vi "Read Save_.vi"(8 "error in (no error)":errorcluster, 11 "Save Data MSG in":refnum<class "Save Data MSG.lvclass">) -> (0 "error out":errorcluster, 2 "Save?":bool, 3 "Save Data MSG out":refnum<class "Save Data MSG.lvclass">)   [LabVIEW 2014, in "Controller.lvlib" / "Save Data MSG.lvclass"]
uses:
  Save Data MSG.lvclass
  Save Data MSG.lvclass/Save Data MSG.ctl
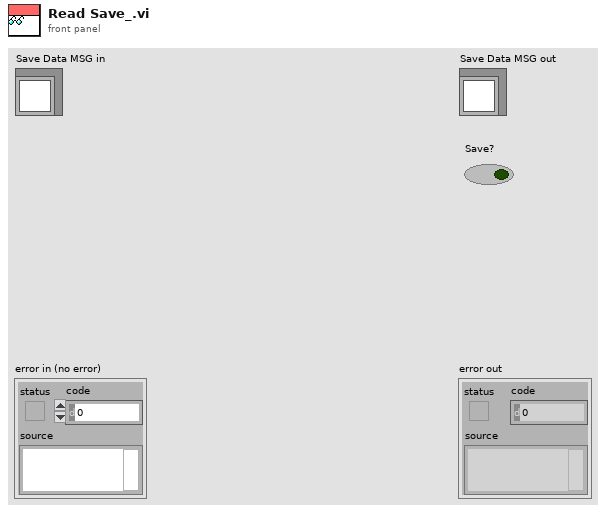
[diagram p1: front panel]
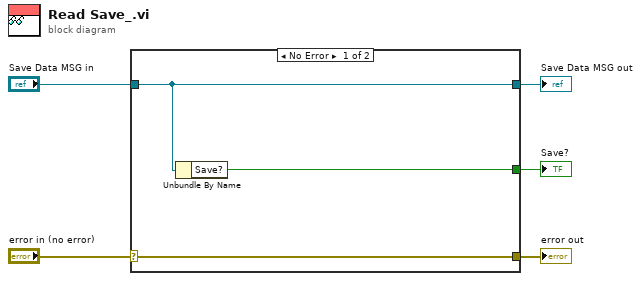
[diagram p0: block diagram]
diagram:
  n1 = case shown="No Error" "error in (no error)" {
    selector: "error in (no error)" -> [w8 w9]
    tunnel: [w8 w9] -> w4
    tunnel: [w7 w10] -> w2
    tunnel: "Save Data MSG in" -> [w7 w10]
    tunnel: [w6 _] -> w1
    frame No Error {
      n2 = Unbundle By Name(w7) -> ("Save?"=w6:bool)
    }
    frame Error {
    }
  }
  "error out" <- w4
  "Save Data MSG out" <- w2
  "Save?" <- w1
